vi "command engine update FIFOs after commands.vi"(8 "error out":errorcluster, 9 "State Variables in":T12, 10 "Parameters in":T1 {"Compiled"."External Channels"."Channels" format="%.0x"; "Compiled"."External Channels"."Triggers" format="%.0x"}, 11 "Global Variables":T15) -> (0 "error out":errorcluster, 1 "State Variables out":T12, 2 "Parameters out":T1 {"Compiled"."External Channels"."Channels" format="%.0x"; "Compiled"."External Channels"."Triggers" format="%.0x"}, 3 "Global Variables out":T15)   [LabVIEW 2015, in "Instrument Addon Engine.lvlib"]
uses:
  Instrument Addon Engine.lvlib
  Types/Commands RT Configuration Cluster.ctl
  Protocols.lvlibp/Protocol Parent/Protocol Parent.lvclass
  Shared/Types/Compiled Settings.ctl
  Shared/Types/Command Parameters.ctl
  Shared/Types/Linked Channel Cluster.ctl
  Shared/Types/Response RT Configuration Cluster.ctl
  Shared/Types/Response Parameters.ctl
  Shared/Types/Response Wait Type.ctl
  Shared/Types/Message Parameters.ctl
  Shared/Types/Message Generation Type.ctl
  Shared/Types/External Trigger Refs.ctl
  <vilib>/NI Veristand/Custom Device API/Data Reference.ctl
  Protections.lvlibp/Parent Protection/Protection.lvclass
  Types/command engine global variables.ctl
  <vilib>/NI/AMC/Message Queue.ctl
  <vilib>/NI/AMC/Message.ctl
  <vilib>/NI/Tools/Keyed Array/KeyedArray.ctl
  Types/Engine State Variables.ctl
  <vilib>/NI/NI VeriStand Inline Async API/_VS Inline Async API/Process/Process.lvclass
  Types/TCP Refs.ctl
  <vilib>/NI/STM/Connection Manager/TCP/Advanced/TCP Connection Manager Reference.ctl
  <vilib>/NI/STM/Connection Manager/TCP/Advanced/TCP Connection Manager State Variables.ctl
  <vilib>/NI/STM/TCP/TCP Connection Info.ctl
  <vilib>/NI/STM/SubVIs/MetaDataElement.ctl
  <vilib>/NI/STM/Connection Manager/TCP/TCP Connection Properties.ctl
  <vilib>/NI/NI VeriStand Inline Async API/_Data Access Engine/Access Type Classes/Write/Write.lvclass
  <vilib>/NI/NI VeriStand Inline Async API/_Data Access Engine/Access Type Classes/Read/Read.lvclass
  <vilib>/NI/NI VeriStand Inline Async API/_Data Access Engine/Access Type Classes/ReadWrite/ReadWrite.lvclass
  <vilib>/NI/NI VeriStand Inline Async API/_Data Access Engine/Access Type Classes/ReadWrite/ReadWrite.lvclass/ReadWrite.ctl
  <vilib>/NI/NI VeriStand Inline Async API/_Data Access Engine/Access Type Classes/Write/Write.lvclass/Write.ctl
  <vilib>/NI/NI VeriStand Inline Async API/_Data Access Engine/Data Access Engine/Methods/Write.Data.vi
  <vilib>/NI/NI VeriStand Inline Async API/_Data Access Engine/Data Access Engine/Methods/ReadWrite.Data.Reset.vi
  <vilib>/NI/NI VeriStand Inline Async API/_Data Access Engine/Access Type Classes/Write/Write.ProcessData.vi
  <vilib>/NI/NI VeriStand Inline Async API/_Data Access Engine/Access Type Classes/ReadWrite/ReadWrite.ProcessData.Reset.vi
  <vilib>/NI/NI VeriStand Inline Async API/_Data Access Engine/Data Access Engine/Data Access Engine.lvclass
  Shared/Instrument Addon Shared.lvlib
  <vilib>/NI VeriStand/Custom Device API/Custom Device API.lvlib
  <vilib>/NI/Tools/Keyed Array/Tools_KeyedArray.lvlib
  <vilib>/NI/AMC/AMC.lvlib
  <vilib>/NI/STM/NI STM.lvlib
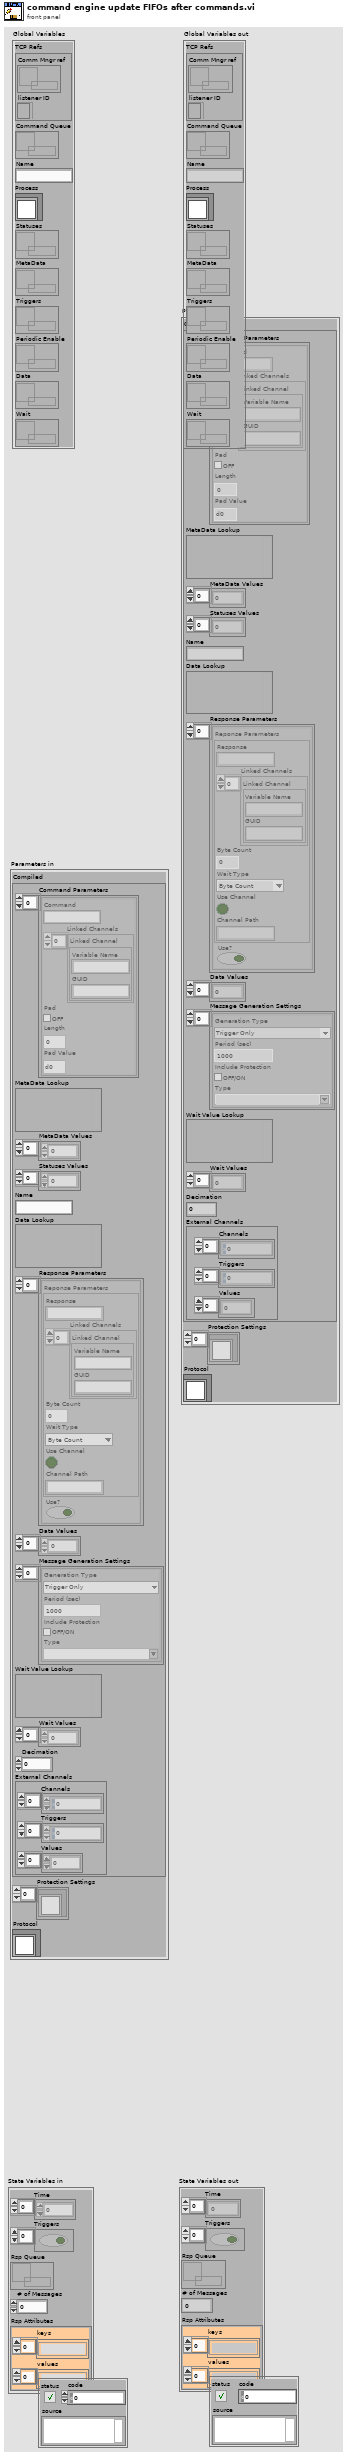
[diagram p1: front panel]
types:
  T1 = typedef "Instrument Addon Engine.lvlib/Commands RT Configuration Cluster.ctl" = cluster{"Compiled":T2, "Protection Settings":refnum<class "Protection.lvclass">[], "Protocol":refnum<class "Protocol Parent.lvclass">}
  T2 = typedef "Instrument Addon Shared.lvlib/Compiled Settings.ctl" = cluster{"Command Parameters":T3[], "MetaData Lookup":variant, "MetaData Values":dbl[], "Statuses Values":dbl[], "Name":string, "Data Lookup":variant, "Response Parameters":T5[], "Data Values":dbl[], "Message Generation Settings":T8[], "Wait Value Lookup":variant, "Wait Values":dbl[], "Decimation":u32, "External Channels":T10}
  T3 = typedef "Instrument Addon Shared.lvlib/Command Parameters.ctl" = cluster{"Command":string, "Linked Channels":T4[], "Pad":bool, "Length":u32, "Pad Value":u8}
  T4 = typedef "Instrument Addon Shared.lvlib/Linked Channel Cluster.ctl" = cluster{"Variable Name":string, "GUID":string}
  T5 = typedef "Instrument Addon Shared.lvlib/Response RT Configuration Cluster.ctl" = cluster{"Reponse Parameters":T6, "Use?":bool}
  T6 = typedef "Instrument Addon Shared.lvlib/Response Parameters.ctl" = cluster{"Response":string, "Linked Channels":T4[], "Type Value":dbl, "Wait Type":T7, "Use Channel":bool, "Channel Path":string}
  T7 = typedef "Instrument Addon Shared.lvlib/Response Wait Type.ctl" = enum16{"Byte Count", "Wait sec"}
  T8 = typedef "Instrument Addon Shared.lvlib/Message Parameters.ctl" = cluster{"Generation Type":T9, "Period":dbl, "Include Protection":bool, "Type":string}
  T9 = typedef "Instrument Addon Shared.lvlib/Message Generation Type.ctl" = enum16{"Trigger Only", "Periodic & Trigger"}
  T10 = typedef "Instrument Addon Shared.lvlib/External Trigger Refs.ctl" = cluster{"Channels":T11[], "Triggers":T11[], "Values":dbl[]}
  T11 = typedef "Custom Device API.lvlib/Data Reference.ctl" = i32
  T12 = typedef "Instrument Addon Engine.lvlib/command engine global variables.ctl" = cluster{"Time":u32[], "Triggers":bool[], "Rsp Queue":T13, "# of Messages":i32, "Rsp Attributes":T14}
  T13 = typedef "AMC.lvlib/Message Queue.ctl" = refnum<queue>
  T14 = typedef "Tools_KeyedArray.lvlib/KeyedArray.ctl" = cluster{"keys":string[], "values":string[]}
  T15 = typedef "Instrument Addon Engine.lvlib/Engine State Variables.ctl" = cluster{"TCP Refs":T16, "Command Queue":T13, "Name":string, "Process":refnum<class "Process.lvclass">, "Statuses":refnum<data-value>, "MetaData":refnum<data-value>, "Triggers":refnum<data-value>, "Periodic Enable":refnum<data-value>, "Data":refnum<data-value>, "Wait":refnum<data-value>}
  T16 = typedef "Instrument Addon Engine.lvlib/TCP Refs.ctl" = cluster{"Comm Mngr ref":T17, "listener ID":refnum<k5>}
  T17 = typedef "TCP Connection Manager Reference.ctl" = refnum<data-value>
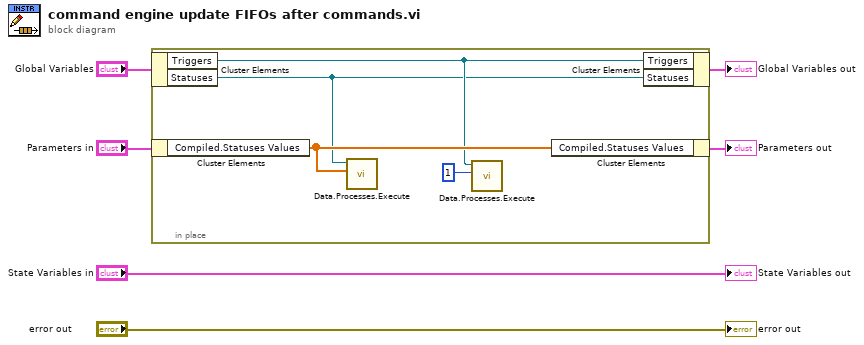
[diagram p0: block diagram]
diagram:
  n1 = in-place {
    n2 = in-place-cluster #1("Global Variables") -> ("Triggers"=w8:refnum<data-value>, "Statuses"=w7:refnum<data-value>)
    n3 = in-place-cluster #2("Parameters in") -> ("Compiled.Statuses Values"=w9:dbl[])
    n4 = call-poly <vilib>:"Data.Processes.Execute.vi"("Values"=w9, "Ref"=w7) -> ()  [unwired: 9 in, 1 out]
    n5 = call-poly <vilib>:"Data.Processes.Execute.vi"("timeout ms"=1, "Ref"=w8) -> ()  [unwired: 8 in, 2 out]
    n6 = in-place-cluster #2("Compiled.Statuses Values"=w9) -> (→"Parameters out":T1)
    n7 = in-place-cluster #1("Triggers"=w8, "Statuses"=w7) -> (→"Global Variables out":T15)
  }
  "State Variables out" <- "State Variables in"
  "error out" <- "error out"
